vi "Format Event Timing Captures into Table.vi"(11 "Captures":T1[](array[typedef])) -> (3 "Table":string[][](array[string]))   [LabVIEW 2013, in "Engine Simulation Toolkit System Explorer.lvlib"]
uses:
  Engine Simulation Toolkit System Explorer.lvlib
  Event Timing Capture.ctl
  Event Reference Angle Selection.ctl
  Shared/Constants and GUIDs.vi
  Shared/Engine Simulation Toolkit Shared.lvlib
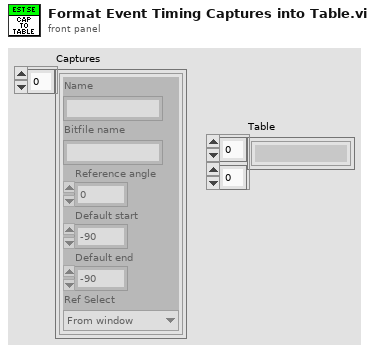
[diagram p1: front panel]
types:
  T1 = typedef "Engine Simulation Toolkit System Explorer.lvlib/Event Timing Capture.ctl" = cluster{"Name":string, "Bitfile name":string, "Reference angle":dbl, "Default start":dbl, "Default end":dbl, "Ref Select":T2}
  T2 = typedef "Engine Simulation Toolkit System Explorer.lvlib/Event Reference Angle Selection.ctl" = enum16{"From window", "Custom"}
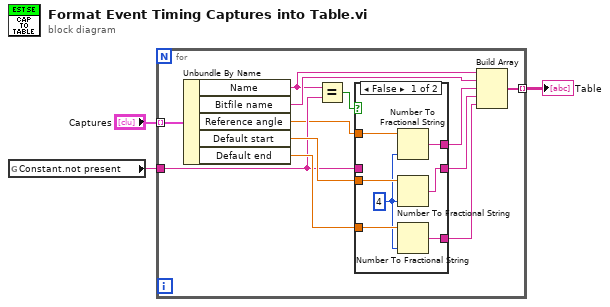
[diagram p0: block diagram]
diagram:
  n1 = global read "Constants and GUIDs.vi" "Constant.not present"() -> (w1:string)
  n2 = for {
    tunnel: "Captures" -> [w15] mode=indexing
    tunnel: [w14] -> w2 mode=indexing
    tunnel: w1 -> [w6]
    n3 = Unbundle By Name(w15) -> ("Name"=w10:string, "Bitfile name"=w13:string, "Reference angle"=w5:dbl, "Default start"=w7:dbl, "Default end"=w12:dbl)
    n4 = Equal?(x=w10, y=w6) -> (x = y?=w9:bool)
    n5 = case shown="False" w9 {
      tunnel: w12 -> [w19 _]
      tunnel: [w20 w23] -> w11
      tunnel: [w17 w23] -> w8
      tunnel: w7 -> [w21 _]
      tunnel: w6 -> [_ w23]
      tunnel: w5 -> [w22 _]
      tunnel: [w16 w23] -> w4
      frame False {
        w18 = i16 4 ("precision (6)")
        n6 = Number To Fractional String(number=w22, precision (6)=w18) -> (F-format string=w16:string)  [unwired: 2 in]
        n7 = Number To Fractional String(number=w21, precision (6)=w18) -> (F-format string=w17:string)  [unwired: 2 in]
        n8 = Number To Fractional String(number=w19, precision (6)=w18) -> (F-format string=w20:string)  [unwired: 2 in]
      }
      frame True {
      }
    }
    n9 = Build Array(w10, w13, w4, w8, w11) -> (w14:string[])
  }
  "Table" <- w2
